vi "PotentialDivider.vi"(11 "Data in":dbl[](array[numeric])) -> (3 "Data out":dbl[](array[numeric]))   [LabVIEW 2020]
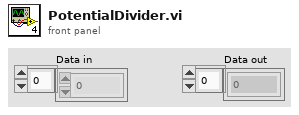
[diagram p1: front panel]
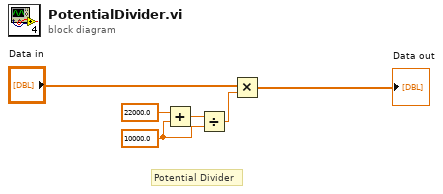
[diagram p0: block diagram]
diagram:
  w2 = 10000.0 ("x+y")
  # "Potential Divider"
  n1 = Add(x=22000.0 ("y"), y=w2) -> (x+y=w1:dbl)
  n2 = Divide(x=w1, y=w2) -> (x/y=w4:dbl)
  n3 = Multiply(x="Data in", y=w4) -> (x*y=→"Data out":dbl[])
